vi "ST5 Load Act .vi"(8 "error in (no error)":errorcluster, 11 "Actuator Settings":string) -> (0 "error out":errorcluster, 1 "Résolution Pas":dbl, 2 "Facteur Pas":dbl=1500.0, 3 "Actuator names":string[](array[string]), 4 "Unit Strings":string[](array[string]), 5 "Units":u16, 6 "Facteur Dir":bool, 7 "Idle Current(A)":dbl)   [LabVIEW 2019]
doc: "Use this template to build a VI to use as a subVI."
uses:
  <vilib>/Utility/config.llb/Read Key (Boolean).vi
  <vilib>/Utility/config.llb/Read Key (String).vi
  <vilib>/Utility/config.llb/Read Key (I32).vi
  <vilib>/Utility/config.llb/Read Key (Double).vi
  <vilib>/Utility/config.llb/NI_LVConfig.lvlib
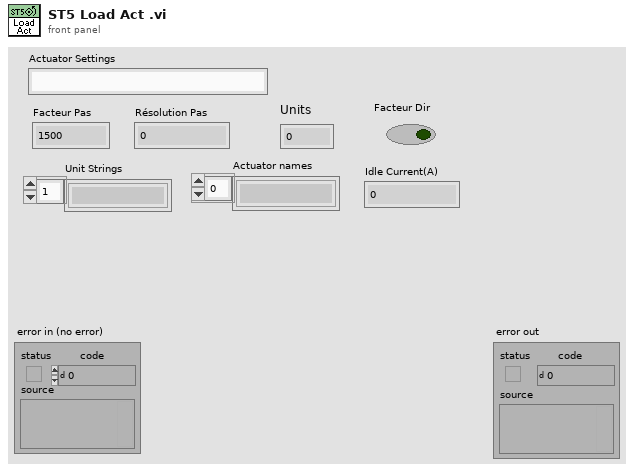
[diagram p1: front panel]
types:
  T1 = typedef "NI_LVConfig.lvlib/Config Data RefNum.ctl" = refnum<k1>
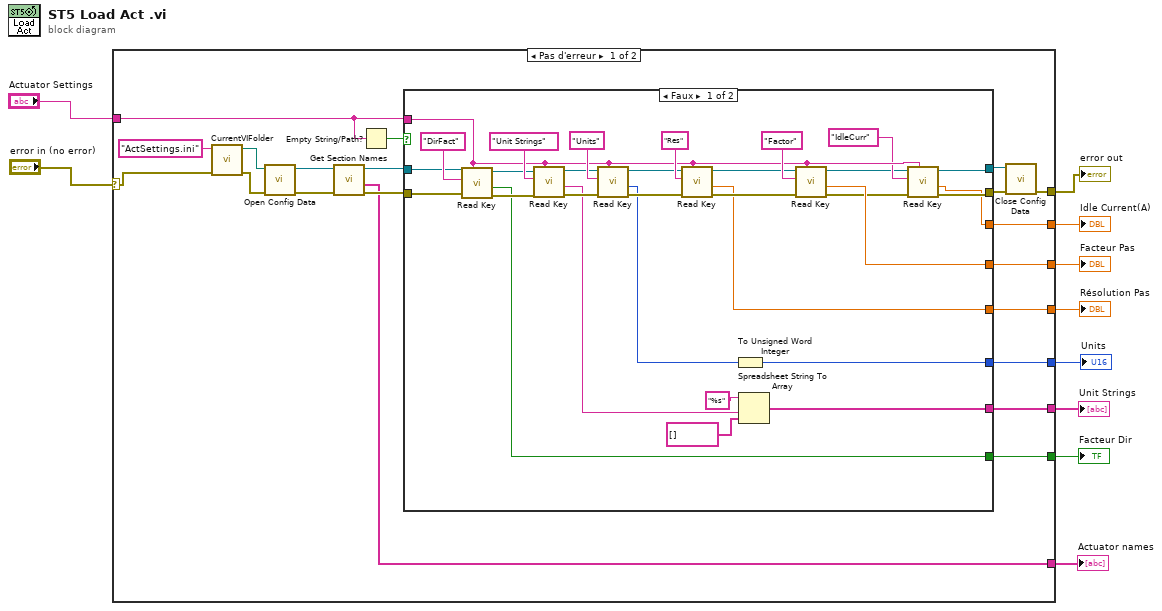
[diagram p0: block diagram]
diagram:
  n1 = case shown="Pas d'erreur" "error in (no error)" {
    selector: "error in (no error)" -> [w28 w64]
    tunnel: [w24 w64] -> w9
    tunnel: "Actuator Settings" -> [w12 _]
    tunnel: [w19 _] -> w7
    tunnel: [w18 _] -> w6
    tunnel: [w16 _] -> w5
    tunnel: [w17 _] -> w4
    tunnel: [w15 _] -> w3
    tunnel: [w14 _] -> w2
    tunnel: [w11 _] -> w1
    frame No Error {
      n2 = call <userlib>:"CurrentVIFolder.vi"("error in (no error)"=w28, "NomFichier"="ActSettings.ini") -> ("error out"=w27:errorcluster, "Chemin"=w30:path)  [unwired: 7 in, 1 out]
      n3 = call <vilib>:"Open Config Data.vi"("error in (no error)"=w27, "configuration file path"=w30) -> ("error out"=w26:errorcluster, "refnum"=w21:T1)  [unwired: 7 in, 1 out]
      n4 = call <vilib>:"Get Section Names.vi"("error in (no error)"=w26, "refnum"=w21) -> ("error out"=w22:errorcluster, "section names"=w19:string[], "refnum out"=w20:T1)  [unwired: 7 in]
      n5 = Empty String/Path?(string/path=w12) -> (empty?=w13:bool)
      n6 = case shown="Faux" w13 {
        tunnel: [w34 w62] -> w25
        tunnel: [w31 w63] -> w23
        tunnel: w12 -> [w37 _]
        tunnel: w22 -> [w46 w62]
        tunnel: w20 -> [w45 w63]
        tunnel: [w44 _] -> w18
        tunnel: [w41 _] -> w17
        tunnel: [w40 _] -> w16
        tunnel: [w39 _] -> w15
        tunnel: [w38 _] -> w14
        tunnel: [w33 _] -> w11
        frame False {
          n7 = call-poly <vilib>:"Read Key.vi"("section"=w37, "error in (no error)"=w46, "key"="DirFact" ("section"), "refnum"=w45) -> ("error out"=w59:errorcluster, "value"=w44:bool, "refnum out"=w58:T1)  [unwired: 4 in, 1 out]
          n8 = call-poly <vilib>:"Read Key.vi"("section"=w37, "error in (no error)"=w59, "key"="Unit Strings", "refnum"=w58) -> ("error out"=w57:errorcluster, "value"=w43:string, "refnum out"=w54:T1)  [unwired: 4 in, 1 out]
          n9 = call-poly <vilib>:"Read Key.vi"("section"=w37, "error in (no error)"=w57, "key"="Units", "refnum"=w54) -> ("error out"=w52:errorcluster, "value"=w42:i32, "refnum out"=w51:T1)  [unwired: 4 in, 1 out]
          n10 = call-poly <vilib>:"Read Key.vi"("section"=w37, "error in (no error)"=w52, "key"="Res", "refnum"=w51) -> ("error out"=w49:errorcluster, "value"=w39:dbl, "refnum out"=w48:T1)  [unwired: 4 in, 1 out]
          n11 = To Unsigned Word Integer(number=w42) -> (unsigned 16bit integer=w40:u16)
          n12 = Spreadsheet String To Array(format string="%s", spreadsheet string=w43, array type (2D Dbl)=string[] []) -> (array=w41:string[])  [unwired: 1 in]
          n13 = call-poly <vilib>:"Read Key.vi"("section"=w37, "error in (no error)"=w49, "key"="Factor", "refnum"=w48) -> ("error out"=w35:errorcluster, "value"=w38:dbl, "refnum out"=w32:T1)  [unwired: 4 in, 1 out]
          n14 = call-poly <vilib>:"Read Key.vi"("section"=w37, "error in (no error)"=w35, "key"="IdleCurr", "refnum"=w32) -> ("error out"=w34:errorcluster, "value"=w33:dbl, "refnum out"=w31:T1)  [unwired: 4 in, 1 out]
        }
        frame True {
        }
      }
      n15 = call <vilib>:"Close Config Data.vi"("error in (no error)"=w25, "refnum"=w23) -> ("error out"=w24:errorcluster)  [unwired: 8 in, 1 out]
    }
    frame Error {
    }
  }
  "error out" <- w9
  "Facteur Pas" <- w2
  "Résolution Pas" <- w3
  "Units" <- w5
  "Facteur Dir" <- w6
  "Unit Strings" <- w4
  "Actuator names" <- w7
  "Idle Current(A)" <- w1
